vi "FTW-Ether-SpawnNewActor-Refnum.vi"(5 "Configuration":string="{\n  \"Identity\": \"ActorName\",\n  \"DebugEnableInboxLogging\": false,\n  \"DebugEnableJobLogging\": false,\n  \"InboxAddress\": \"inproc://*\",\n  \"DebugShowPanel\": false\n}", 7 "Actor VI Refnum":refnum<vi>, 9 "Timeout":i32=1000 format="%dmsec", 11 "error in":errorcluster) -> (4 "FTW Actor Connector":refnum<class "FTW-ActorConnector.lvclass">, 6 "Initialized Response":string, 8 "Instance Inbox Address":string, 15 "error out":errorcluster)   [LabVIEW 2015, in "FTW-Ether.lvclass"]
doc: "This is the spawn new actor that was used for a while. It lacks the minimum strict inputs required to launch an actor."
uses:
  FTW-Ether.lvclass
  Connector/FTW-ActorConnector.lvclass
panel:
  # "Inputs"
  # "Outputs"
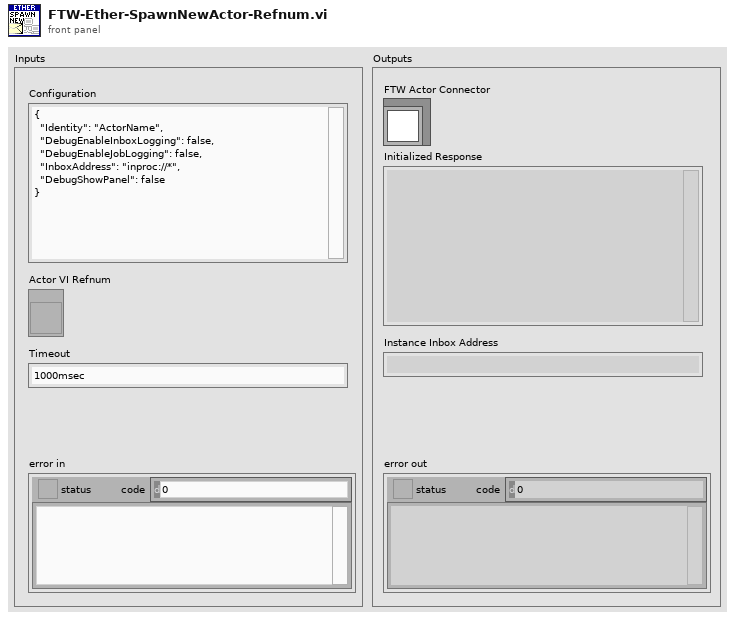
[diagram p1: front panel]
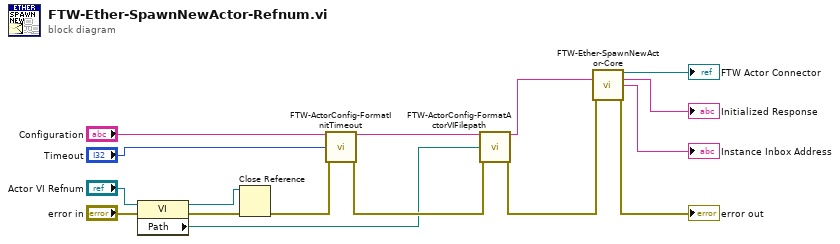
[diagram p0: block diagram]
diagram:
  n1 = property class="VI"(reference="Actor VI Refnum", error in="error in") -> (reference out=w2:refnum<vi>, error out=w5:errorcluster, "Path"=w1:path)
  n2 = Close Reference(reference=w2, error in (no error)=w5) -> (error out=w3:errorcluster)
  n3 = call "FTW-ActorConfig-FormatInitTimeout.vi"("FTW Config String In"="Configuration", "Init Timeout"="Timeout", "error in"=w3) -> ("FTW Config String"=w9:string, "error out"=w7:errorcluster)  [unwired: 11 in]
  n4 = call "FTW-ActorConfig-FormatActorVIFilepath.vi"("FTW Config String In"=w9, "Actor VI Filepath"=w1, "error in"=w7) -> ("FTW Config String"=w8:string, "error out"=w6:errorcluster)  [unwired: 11 in]
  n5 = call "FTW-Ether-SpawnNewActor-Core.vi"("Configuration"=w8, "error in"=w6) -> ("FTW Actor Connector"=→"FTW Actor Connector":refnum<class "FTW-ActorConnector.lvclass">, "Initialized Response"=→"Initialized Response":string, "Instance Inbox Address"=→"Instance Inbox Address":string, "error out"=→"error out":errorcluster)  [unwired: 10 in]
